vi "magnet initialize.vi"(8 "error in (no error)":errorcluster) -> (0 "error out":errorcluster)   [LabVIEW 2016]
uses:
  config.vi
panel:
  out "Numeric":dbl format="%#_13g"
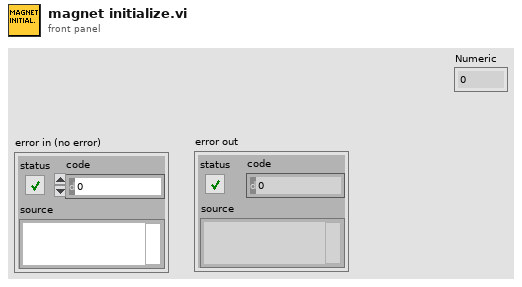
[diagram p1: front panel]
types:
  T1 = cluster{"GPIB address":i16, "GPIB bus":i16, "connection ID":refnum<k5>, "IP":string, "Active Comm Interface":u16, "Serial Port":refnum<visa-resource-name>, "Programmer Type":u16}
  T2 = cluster{"error":bool, "code":i32, "source":string}
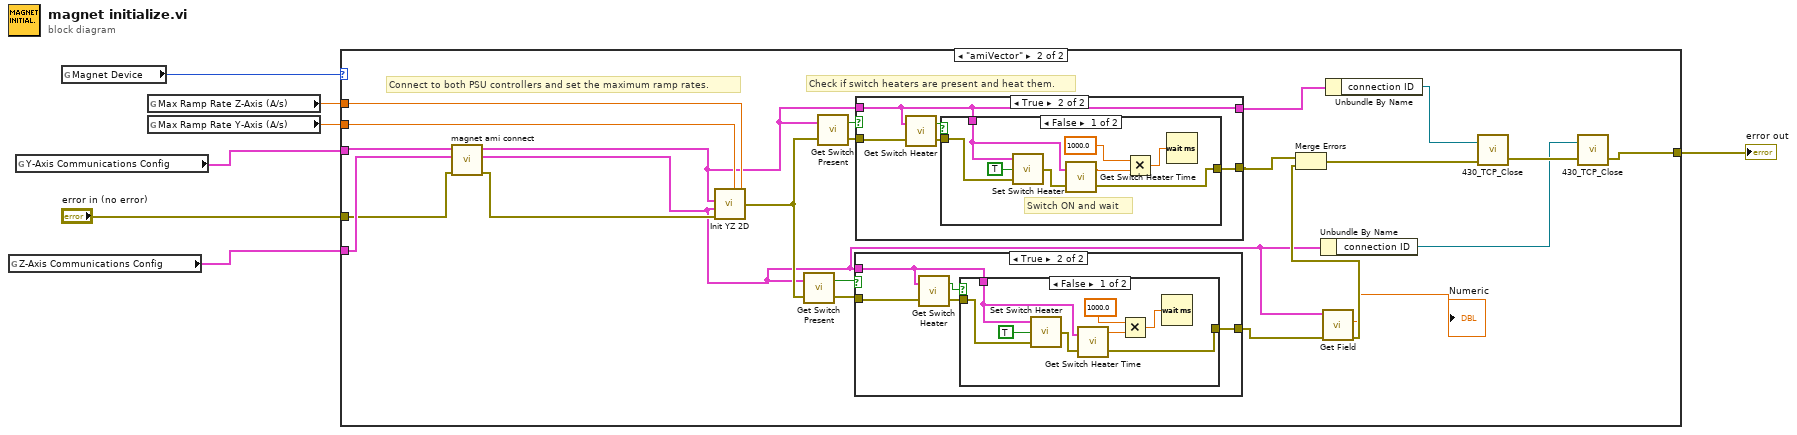
[diagram p0: block diagram]
diagram:
  n1 = global read "config.vi" "Z-Axis Communications Config"() -> (w5:T1)
  n2 = global read "config.vi" "Y-Axis Communications Config"() -> (w4:T1)
  n3 = global read "config.vi" "Magnet Device"() -> (w7:enum16{"ips120", "amiVector"})
  n4 = global read "config.vi" "Max Ramp Rate Z-Axis (A/s)"() -> (w2:dbl)
  n5 = global read "config.vi" "Max Ramp Rate Y-Axis (A/s)"() -> (w3:dbl)
  n6 = case shown="\"amiVector\"" w7 {
    tunnel: "error in (no error)" -> [w8 w17]
    tunnel: w5 -> [_ w18]
    tunnel: w4 -> [_ w19]
    tunnel: w3 -> [_ w30]
    tunnel: w2 -> [_ w31]
    tunnel: [w8 w24] -> w1
    frame "ips120", Default {
    }
    frame "amiVector" {
      # "Check if switch heaters are present and heat them."
      # "Connect to both PSU controllers and set the maximum ramp rates."
      n7 = call "magnet ami connect.vi"("error in (no error)"=w17, "Z-Axis Communications Config"=w18, "Y-Axis Communications Config"=w19) -> ("error out"=w16:errorcluster, "Z-Axis Communications Config Out"=w10:T1, "Y-Axis Communications Config Out"=w15:T1)  [unwired: 6 in]
      n8 = call "Init YZ 2D.vi"("Max Ramp Rate Z-axis"=w31, "Max Ramp Rate Y-axis"=w30, "error in"=w16, "Z-Axis Communications Config"=w10, "Y-Axis Communications Config"=w15) -> ("error out"=w25:T2)  [unwired: 5 in]
      n9 = call "Get Switch Present.vi"("error in"=w25, "Communications Config"=w10) -> ("error out"=w29:T2, "Switch Present?"=w28:bool)
      n10 = call "Get Switch Present.vi"("error in"=w25, "Communications Config"=w15) -> ("error out"=w27:T2, "Switch Present?"=w26:bool)
      n11 = case shown="True" w28 {
        tunnel: w29 -> [w48 w51]
        tunnel: w10 -> [_ w50]
        tunnel: [w48 w49] -> w12
        frame False {
        }
        frame True {
          n12 = call "Get Switch Heater.vi"("error in"=w51, "Communications Config"=w50) -> ("error out"=w53:T2, "Switch Heater Indicator"=w52:bool)
          n13 = case shown="False" w52 {
            tunnel: w53 -> [w60 w62]
            tunnel: w50 -> [w56 _]
            tunnel: [w54 w62] -> w49
            frame False {
              n14 = call "Set Switch Heater.vi"("error in"=w60, "Switch Heater Control"=TRUE, "Communications Config"=w56) -> ("error out"=w55:T2)
              n15 = call "Get Switch Heater Time.vi"("error in"=w55, "Communications Config"=w56) -> ("error out"=w54:T2, "Switch Heating Time (secs)"=w57:dbl)
              n16 = Multiply(x=1000.0 ("y"), y=w57) -> (x*y=w59:dbl)
              n17 = Wait (ms)(milliseconds to wait=w59) -> ()  [unwired: 1 out]
            }
            frame True {
            }
          }
        }
      }
      n18 = case shown="True" w26 {
        tunnel: w27 -> [w32 w37]
        tunnel: w15 -> [w33 w38]
        tunnel: [w33 w38] -> w22
        tunnel: [w32 w34] -> w13
        frame False {
        }
        frame True {
          n19 = call "Get Switch Heater.vi"("error in"=w37, "Communications Config"=w38) -> ("error out"=w36:T2, "Switch Heater Indicator"=w35:bool)
          n20 = case shown="False" w35 {
            tunnel: w36 -> [w45 w47]
            tunnel: [w41 w47] -> w34
            tunnel: w38 -> [w39 _]
            frame False {
              # "Switch ON and wait"
              n21 = call "Set Switch Heater.vi"("error in"=w45, "Switch Heater Control"=TRUE, "Communications Config"=w39) -> ("error out"=w40:T2)
              n22 = call "Get Switch Heater Time.vi"("error in"=w40, "Communications Config"=w39) -> ("error out"=w41:T2, "Switch Heating Time (secs)"=w42:dbl)
              n23 = Multiply(x=1000.0 ("y"), y=w42) -> (x*y=w44:dbl)
              n24 = Wait (ms)(milliseconds to wait=w44) -> ()  [unwired: 1 out]
            }
            frame True {
            }
          }
        }
      }
      n25 = Unbundle By Name(w10) -> ("connection ID"=w20:refnum<k5>)
      n26 = call "Get Field.vi"("Z-Axis Communications Config"=w10, "error in"=w12) -> ("Field(T)"=→"Numeric":dbl, "error out"=w11:T2)  [unwired: 4 in, 1 out]
      n27 = Merge Errors(w13, w11) -> (w14:errorcluster)
      n28 = Unbundle By Name(w22) -> ("connection ID"=w21:refnum<k5>)
      n29 = call "430_TCP_Close.vi"("error in (no error)"=w14, "connection ID"=w21) -> ("error out"=w23:errorcluster)  [unwired: 1 out]
      n30 = call "430_TCP_Close.vi"("error in (no error)"=w23, "connection ID"=w20) -> ("error out"=w24:errorcluster)  [unwired: 1 out]
    }
  }
  "error out" <- w1
